vi "Get MB session in.vi"(11 "THM-V6数字型温湿度 in":refnum<class "THM-V6数字型温湿度.lvclass">) -> (2 "MB Serial Master:MB_Master":refnum<class "MB_Master.lvclass">, 3 "THM-V6数字型温湿度 out":refnum<class "THM-V6数字型温湿度.lvclass">)   [LabVIEW 2016, in "THM-V6数字型温湿度.lvlib" / "THM-V6数字型温湿度.lvclass"]
uses:
  <vilib>/Plasmionique/MB Master/MB_Master/MB_Master.lvclass
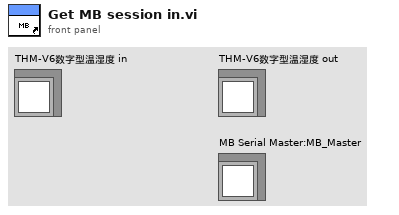
[diagram p1: front panel]
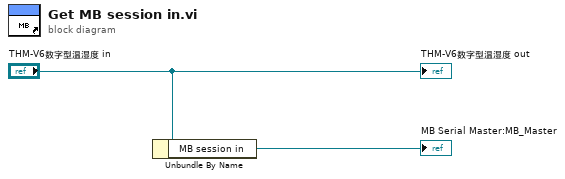
[diagram p0: block diagram]
diagram:
  n1 = Unbundle By Name("THM-V6数字型温湿度 in") -> ("MB session in"=→"MB Serial Master:MB_Master":refnum<class "MB_Master.lvclass">)
  "THM-V6数字型温湿度 out" <- "THM-V6数字型温湿度 in"
